vi "OAT Unfiltered Orbit Plot (Waveform).vi"(0 "waveform X":waveform(dbl), 1 "XY graph Ref":refnum<vi>, 5 "waveform Y":waveform(dbl), 7 "speed profile":T1 {"speed [RPM]" format="%.2f"; "time [s]" format="%.2f"}, 9 "pulse/revolution (1)":i32=1, 11 "error in (no error)":errorcluster, 12 "orbit segment":cluster{"position":dbl, "tach duty":dbl}={"position"=0.0, "tach duty"=0.98} {"tach duty" format="%.2f"; "position" format="%.2f"}, 13 "probe angle":u16(ring) items=["0", "45", "90", "135", "180", "225", "270", "315"]) -> (4 "XY plot value":cluster{"X":dbl[], "Y":dbl[]}[](array[cluster]) {"Y" format="%.2f"; "X" format="%.2f"}, 15 "error out":errorcluster)   [LabVIEW 2017]
doc: "Draws an orbit plot of waveform signals on a XY graph. You can use sampled or resampled waveform signals from proximity transducers. You can use this polymorphic VI to draw an orbit plot of resampled signals or waveform signals. The data types you wire to the <B>resampled signal(X)</B> and <B>resampled signal (Y)</B> inputs determine the polymorphic instance to use."
uses:
  <vilib>/addons/Sound and Vibration/Order Analysis/Tach Process/SubVIs/speed profile.ctl
  <vilib>/Waveform/WDTOps.llb/WDT Get Waveform Subset DBL.vi
  <vilib>/Waveform/WDTOps.llb/WDT Get XY Value DBL.vi
  <vilib>/addons/Sound and Vibration/Order Analysis/Tach Process/SoundVib_TachProcess.lvlib
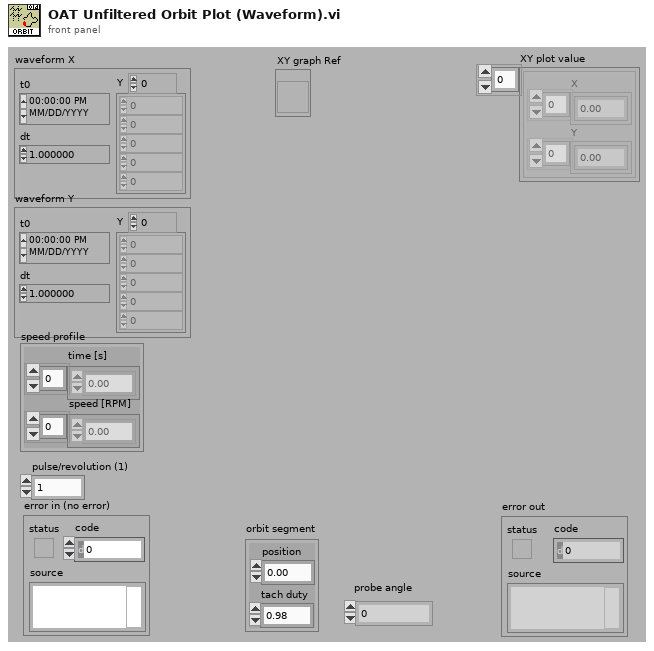
[diagram p1: front panel]
types:
  T1 = typedef "SoundVib_TachProcess.lvlib/speed profile.ctl" = cluster{"time [s]":dbl[], "speed [RPM]":dbl[]}
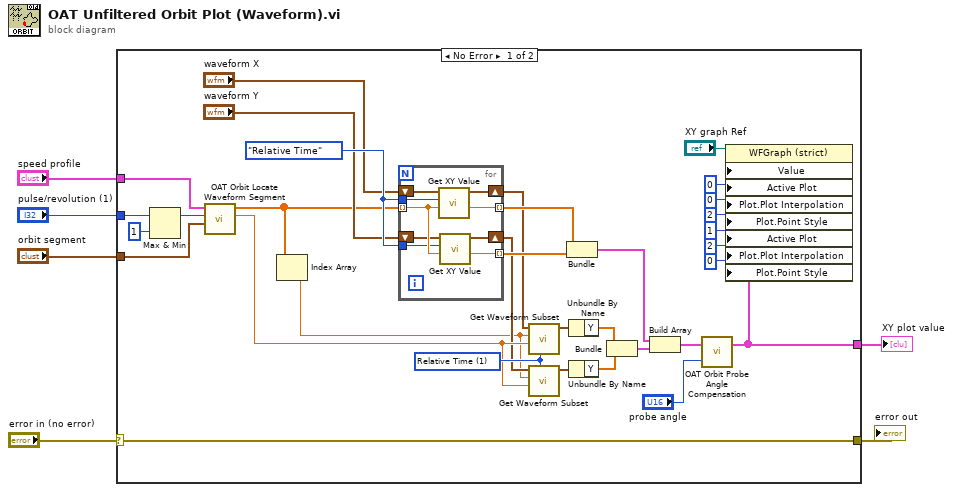
[diagram p0: block diagram]
diagram:
  n1 = case shown="No Error" "error in (no error)" {
    selector: "error in (no error)" -> [w10 w49]
    tunnel: "speed profile" -> [w27 _]
    tunnel: "pulse/revolution (1)" -> [w20 _]
    tunnel: "orbit segment" -> [w15 _]
    tunnel: [w11 _] -> w3
    tunnel: [w10 w49] -> w1
    frame No Error {
      w23 = enum16{"Index", "Relative Time"}."Relative Time" ("mode")
      w39 = u16 1 items=["Index", "Relative Time"] ("Mode")
      n2 = Max & Min(x=w20, y=1) -> (max(x,y)=w9:i32)  [unwired: 1 out]
      n3 = call <vilib>:"OAT Orbit Locate Waveform Segment.vi"("orbit segment"=w15, "pulse/revolution (1)"=w9, "speed profile"=w27) -> ("duration"=w26:dbl, "start points"=w14:dbl[])  [unwired: 6 in, 1 out]
      n4 = Index Array(array=w14) -> (element=w7:dbl)  [unwired: 1 in]
      n5 = for {
        tunnel: w14 -> [w48] mode=indexing
        tunnel: w23 -> [w47]
        tunnel: w23 -> [w46]
        tunnel: [w45] -> w22 mode=indexing
        tunnel: [w44] -> w21 mode=indexing
        shift-right: [w43] -> w18
        shift-left: "waveform X" -> [w42]
        shift-right: [w40] -> w16
        shift-left: "waveform Y" -> [w41]
        n6 = call-poly <vilib>:"Get XY Value.vi"("Y position"=w48, "Y position format"=w47, "waveform in"=w42) -> ("Y value"=w45:dbl, "waveform out"=w43:waveform(dbl))  [unwired: 4 in, 3 out]
        n7 = call-poly <vilib>:"Get XY Value.vi"("Y position"=w48, "Y position format"=w46, "waveform in"=w41) -> ("Y value"=w44:dbl, "waveform out"=w40:waveform(dbl))  [unwired: 4 in, 3 out]
      }
      n8 = call-poly <vilib>:"Get Waveform Subset.vi"("start/duration format"=w39, "duration"=w26, "start samples/time"=w7, "waveform in"=w18) -> ("waveform out"=w38:waveform(dbl))  [unwired: 2 in, 3 out]
      n9 = call-poly <vilib>:"Get Waveform Subset.vi"("start/duration format"=w39, "duration"=w26, "start samples/time"=w7, "waveform in"=w16) -> ("waveform out"=w37:waveform(dbl))  [unwired: 2 in, 3 out]
      n10 = Bundle(w22, w21) -> (w35:cluster{dbl[], dbl[]})  [unwired: 1 in]
      n11 = Unbundle By Name(w38) -> ("Y"=w24:dbl[])
      n12 = Unbundle By Name(w37) -> ("Y"=w25:dbl[])
      n13 = Bundle("Y"=w24, "Y"=w25) -> (w36:cluster{"Y":dbl[], "Y":dbl[]})  [unwired: 1 in]
      n14 = Build Array(w35, w36) -> (w13:cluster{"Y":dbl[], "Y":dbl[]}[])
      n15 = call <vilib>:"OAT Orbit Probe Angle Compensation.vi"("probe angle compensation"="probe angle", "XY plot data in"=w13) -> ("XY plot data out"=w11:cluster{dbl[], dbl[]}[])  [unwired: 1 in]
      n16 = property class="WFGraph (strict)"(reference="XY graph Ref", "Value"=w11, "Active Plot"=u32 0, "Plot.Plot Interpolation"=u8 0, "Plot.Point Style"=u8 2, "Active Plot"=u32 1, "Plot.Plot Interpolation"=u8 2, "Plot.Point Style"=u8 0) -> ()  [unwired: 1 in, 2 out]
    }
    frame Error {
    }
  }
  "error out" <- w1
  "XY plot value" <- w3
